vi "Word_Update_Chart.vi"(0 "Word.InlineShapes":refnum<k7>, 1 "chart data":dbl[][](array[numeric]) format="%.2f", 9 "Chart index":u16, 11 "error in":errorcluster, 12 "column header":string[](array[string]), 13 "row header":string[](array[string])) -> (15 "error out":errorcluster)   [LabVIEW 2010, in "NI_ReportGenerationToolkit.lvlib"]
uses:
  <vilib>/addons/_office/NI_ReportGenerationToolkit.lvlib
panel:
  in  "MS Graph":refnum<k7>
  in  "Graph.Chart":refnum<k7>
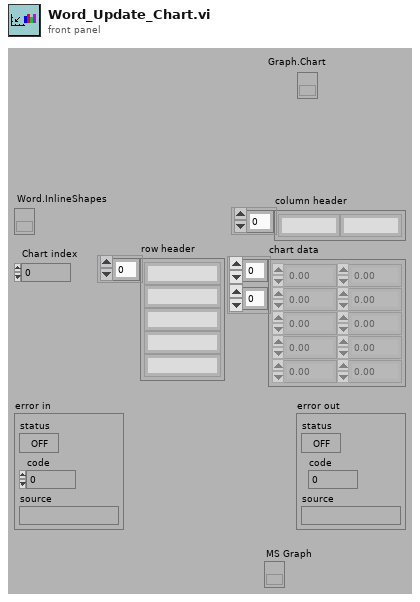
[diagram p1: front panel]
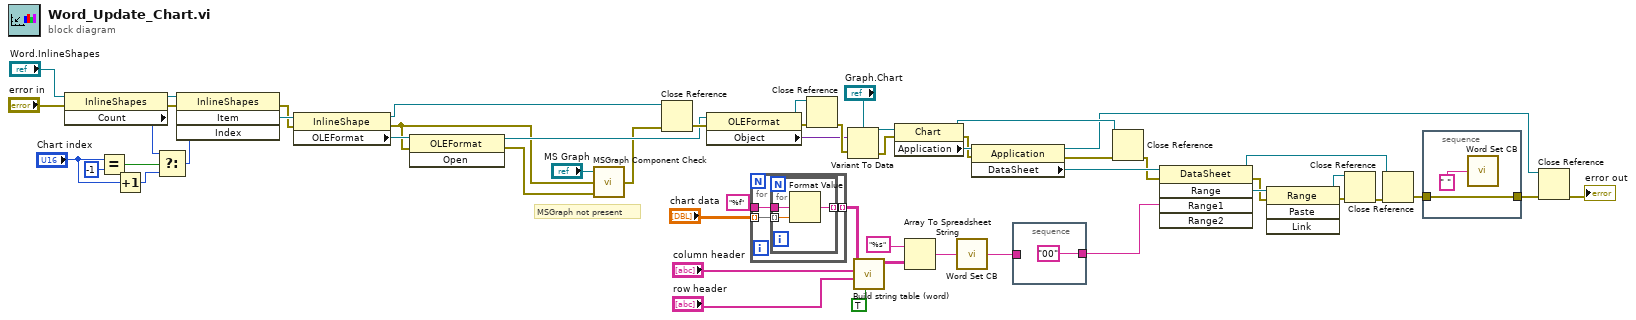
[diagram p0: block diagram]
diagram:
  # "MSGraph not present"
  n1 = property class="InlineShapes"(reference="Word.InlineShapes", error in="error in") -> (reference out=w42:refnum<k7>, error out=w47:errorcluster, "Count"=w34:i32)
  n2 = Equal?(x="Chart index", y=i16 -1) -> (x = y?=w41:bool)
  n3 = Increment(x="Chart index") -> (x+1=w39:u16)
  n4 = Select(t=w34, s=w41, f=w39) -> (s? t:f=w38:i32)
  n5 = invoke class="InlineShapes" method="Item"(reference=w42, error in=w47, "Index"=w38) -> (error out=w43:errorcluster, "Item"=w44:refnum<k7>)  [unwired: 1 in, 2 out]
  n6 = property class="InlineShape"(reference=w44, error in=w43) -> (reference out=w46:refnum<k7>, error out=w4:errorcluster, "OLEFormat"=w9:refnum<k7>)
  n7 = invoke class="OLEFormat" method="Open"(reference=w9, error in=w4) -> (reference out=w8:refnum<k7>, error out=w3:errorcluster)  [unwired: 1 in, 1 out]
  n8 = call <vilib>:"MSGraph Component Check.vi"("error 2"=w3, "error 1"=w4, "MS Graph"="MS Graph") -> ("error out"=w2:errorcluster)
  n9 = Close Reference(reference=w46, error in (no error)=w2) -> (error out=w45:errorcluster)
  n10 = property class="OLEFormat"(reference=w8, error in=w45) -> (reference out=w31:refnum<k7>, error out=w32:errorcluster, "Object"=w33:variant)
  n11 = for {
    tunnel: "chart data" -> [w57] mode=indexing
    tunnel: "%f" -> [w56]
    tunnel: [w55] -> w30 mode=indexing
    n12 = for {
      tunnel: w57 -> [w60] mode=indexing
      tunnel: w56 -> [w59]
      tunnel: [w58] -> w55 mode=indexing
      n13 = Format Value(format string=w59, value (0)=w60) -> (output string=w58:string)  [unwired: 1 out]
    }
  }
  n14 = Close Reference(reference=w31, error in (no error)=w32) -> (error out=w49:errorcluster)
  n15 = Variant To Data(error in=w49, Variant=w33, type="Graph.Chart") -> (error out=w48:errorcluster, data=w53:refnum<k7>)
  n16 = call <vilib>:"Build string table (word).vi"("Graph data?"=TRUE, "row headers"="row header", "column headers"="column header", "text data"=w30) -> ("output table"=w28:string[][])  [unwired: 7 out]
  n17 = property class="Chart"(reference=w53, error in=w48) -> (reference out=w50:refnum<k7>, error out=w51:errorcluster, "Application"=w52:refnum<k7>)
  n18 = Array To Spreadsheet String(array=w28, 3:"%s" ("format string")) -> (spreadsheet string=w7:string)  [unwired: 1 out]
  n19 = call <vilib>:"Word Set CB.vi"("String"=w7) -> ("String 2"=w6:string)
  n20 = property class="Application"(reference=w52, error in=w51) -> (reference out=w11:refnum<k7>, error out=w13:errorcluster, "DataSheet"=w18:refnum<k7>)
  n21 = stacked-sequence {
    tunnel: ["00"] -> w14
    tunnel: w6 -> [_]
    frame #0 {
    }
  }
  n22 = Close Reference(reference=w50, error in (no error)=w13) -> (error out=w17:errorcluster)
  n23 = invoke class="DataSheet" method="Range"(reference=w18, error in=w17, "Range1"=w14) -> (reference out=w20:refnum<k7>, error out=w19:errorcluster, "Range"=w21:refnum<k7>)  [unwired: 2 in, 2 out]
  n24 = invoke class="Range" method="Paste"(reference=w21, error in=w19) -> (reference out=w23:refnum<k7>, error out=w24:errorcluster)  [unwired: 2 in, 2 out]
  n25 = Close Reference(reference=w23, error in (no error)=w24) -> (error out=w22:errorcluster)
  n26 = Close Reference(reference=w20, error in (no error)=w22) -> (error out=w16:errorcluster)
  n27 = stacked-sequence {
    tunnel: w16 -> [w63]
    tunnel: [w63] -> w12
    frame #0 {
      n28 = call <vilib>:"Word Set CB.vi"("String"=" ") -> ()  [unwired: 1 out]
    }
  }
  n29 = Close Reference(reference=w11, error in (no error)=w12) -> (error out=→"error out":errorcluster)
